vi "TestHIL.vi"() -> ()   [LabVIEW 2010]
uses:
  <vilib>/picture/picture.llb/Draw True-Color Pixmap.vi
panel:
  out "Packet Sent":string
  out "Bytes written":i32
  out "Packet Payload":string
  out "bytes read":i32
  out "Counter Send/receive":i16(graph)
  in  "Receiver port number":i32=9002
  in  "Sender port number":i32=9002
  out "KTH  Automatic Control \nTemplates. Test Bi-directional communication \nSerialForwarder-Mote":picture
  # "READ PACKET"
  # "WRITE PACKET"
  # "Communication control"
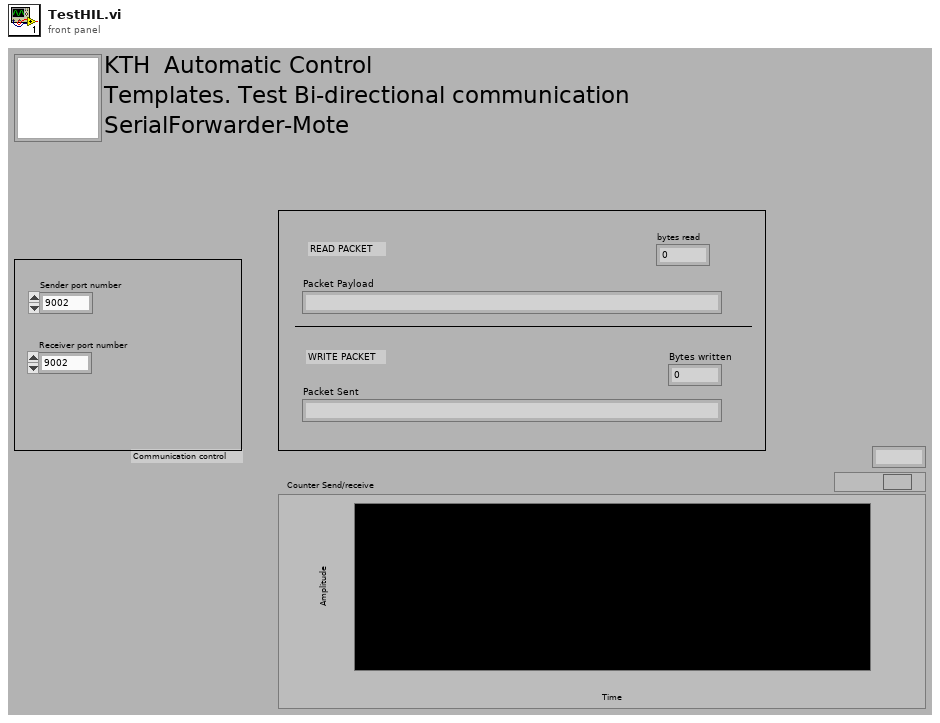
[diagram p1: front panel]
types:
  T1 = typedef "imagedata.ctl" = cluster{"image type":i32, "image depth":i32, "image":u8[], "mask":u8[], "colors":u32[], "Rectangle":cluster{"left":i16, "top":i16, "right":i16, "bottom":i16}}
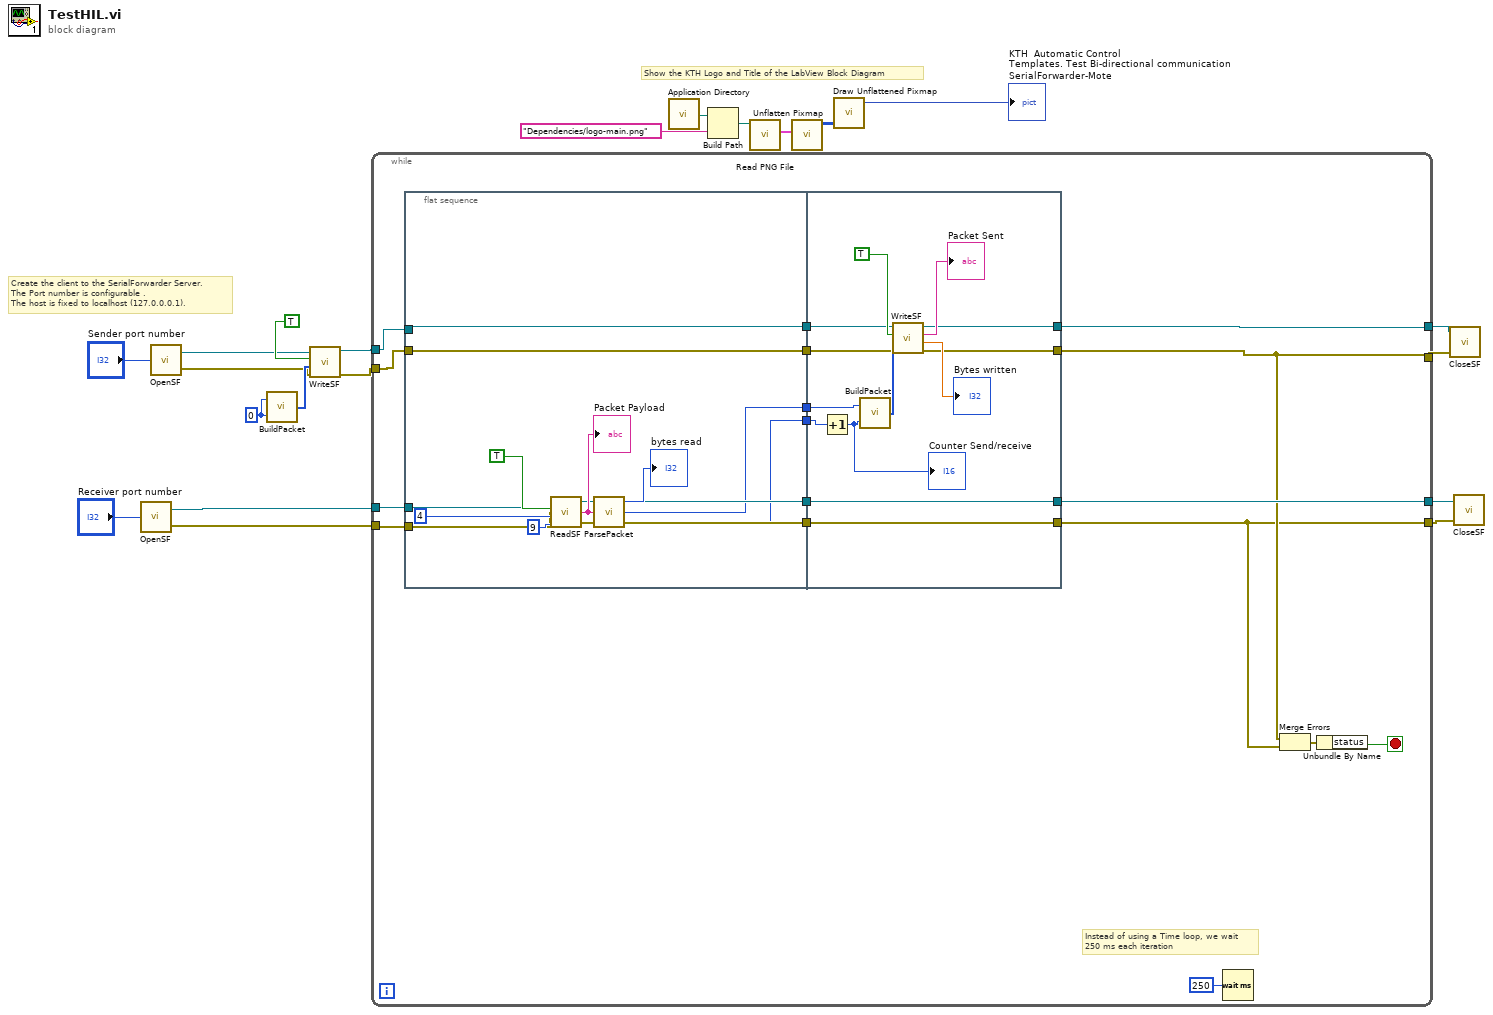
[diagram p0: block diagram]
diagram:
  w2 = i16 0 ("Counter")
  # "Create the client to the SerialForwarder Server.\nThe Port number is configurable . \nThe host is fixed to localhost (127.0.0.0.1)."
  # "Show the KTH Logo and Title of the LabView Block Diagram"
  n1 = call "OpenSF.vi"("Port Number"="Receiver port number") -> ("error out"=w12:errorcluster, "connection ID"=w13:refnum<k5>)
  n2 = call "OpenSF.vi"("Port Number"="Sender port number") -> ("error out"=w4:errorcluster, "connection ID"=w3:refnum<k5>)
  n3 = call "BuildPacket.vi"("Counter"=w2, "Dummy"=w2) -> ("PacketArray"=w6:i32[])
  n4 = call "WriteSF.vi"("error in"=w4, "packet"=w6, "Enablle write"=TRUE ("Enable Write"), "connection ID"=w3) -> ("error out"=w1:errorcluster, "connection ID out"=w5:refnum<k5>)  [unwired: 2 out]
  n5 = while {
    tunnel: w5 -> [w23]
    tunnel: w1 -> [w22]
    tunnel: w13 -> [w32]
    tunnel: w12 -> [w31]
    tunnel: [w34] -> w11
    tunnel: [w27] -> w10
    tunnel: [w30] -> w9
    tunnel: [w26] -> w8
    stop <- w38 stop-if-true
    # "Instead of using a Time loop, we wait \n250 ms each iteration"
    n6 = flat-sequence {
      tunnel: w23 -> [w46]
      tunnel: [w46] -> w35
      tunnel: w22 -> [w45]
      tunnel: [w45] -> w33
      tunnel: w32 -> [w44]
      tunnel: w31 -> [w43]
      tunnel: [w42] -> w29
      tunnel: [w41] -> w28
      tunnel: [w40] -> w25
      tunnel: [w39] -> w24
      tunnel: w35 -> [w60]
      tunnel: [w59] -> w34
      tunnel: [w58] -> w27
      tunnel: w33 -> [w57]
      tunnel: [w56] -> w30
      tunnel: w29 -> [w56]
      tunnel: [w55] -> w26
      tunnel: w28 -> [w55]
      tunnel: w25 -> [w54]
      tunnel: w24 -> [w53]
      frame #0 {
        n7 = call "ReadSF.vi"("connection ID in"=w44, "enabled"=TRUE ("Enable Read"), "bytes to read"=4, "header size"=9 ("bytes to read"), "error in"=w43) -> ("connection ID out"=w42:refnum<k5>, "string"=w50:string, "error out"=w41:errorcluster)
        "Packet Payload" <- w50
        n8 = call "ParsePacket.vi"("data out"=w50) -> ("Counter"=w39:i16, "Dummy"=w40:i16, "Bytes read"=→"bytes read":i32)
      }
      frame #1 {
        n9 = Increment(x=w53) -> (x+1=w52:i16)
        "Counter Send/receive" <- w52
        n10 = call "BuildPacket.vi"("Counter"=w52, "Dummy"=w54) -> ("PacketArray"=w61:i32[])
        n11 = call "WriteSF.vi"("error in"=w57, "packet"=w61, "Enablle write"=TRUE ("Enable Write"), "connection ID"=w60) -> ("error out"=w58:errorcluster, "Bytes written to SF"=→"Bytes written":dbl, "Packet String"=→"Packet Sent":string, "connection ID out"=w59:refnum<k5>)
      }
    }
    n12 = Wait (ms)(milliseconds to wait=u32 250) -> ()  [unwired: 1 out]
    n13 = Merge Errors(w27, w26) -> (w36:errorcluster)
    n14 = Unbundle By Name(w36) -> ("status"=w38:bool)
  }
  n15 = call <vilib>:"Application Directory.vi"() -> ("Application Directory"=w17:path)
  n16 = Build Path(base path=w17, name or relative path="Dependencies/logo-main.png") -> (appended path=w18:path)
  n17 = call <vilib>:"Read PNG File.vi"("path to PNG file"=w18) -> ("image data"=w21:T1)  [unwired: 8 in, 2 out]
  n18 = call <vilib>:"Unflatten Pixmap.vi"("image data"=w21) -> ("24-bit pixmap"=w20:u32[][])  [unwired: 4 in, 6 out]
  n19 = call-poly <vilib>:"Draw Unflattened Pixmap.vi"("data (RGB format)"=w20) -> ("new picture"=→"KTH  Automatic Control \nTemplates. Test Bi-directional communication \nSerialForwarder-Mote":picture)  [unwired: 8 in]
  n20 = call "CloseSF.vi"("error out"=w10, "connection ID"=w11) -> ()  [unwired: 1 in]
  n21 = call "CloseSF.vi"("error out"=w8, "connection ID"=w9) -> ()  [unwired: 1 in]
